vi "TDS RF Power Input Read.vi"(6 "Reference Level (dBm)":dbl, 8 "error in (no error)":errorcluster, 9 "Center Frequency (MHz)":dbl, 10 "Signal InstConfig":string, 11 "Address":string) -> (0 "error out":errorcluster, 3 "Power":dbl)   [LabVIEW 2025, in "Interface Functions.lvlib"]
uses:
  Interface Functions.lvlib
  <vilib>/Utility/error.llb/Trim Whitespace One-Sided.vi
  <instrlib>/Agilent U2000 Series/Agilent U2000 Series.lvlib
panel:
  out "Offset":dbl
  out "Commands":string[](array[string])
  # "RF Power Input Read"
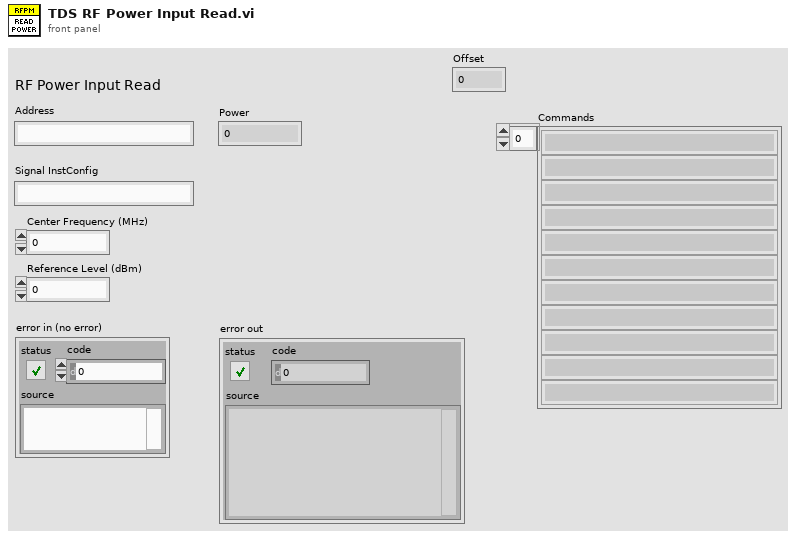
[diagram p1: front panel]
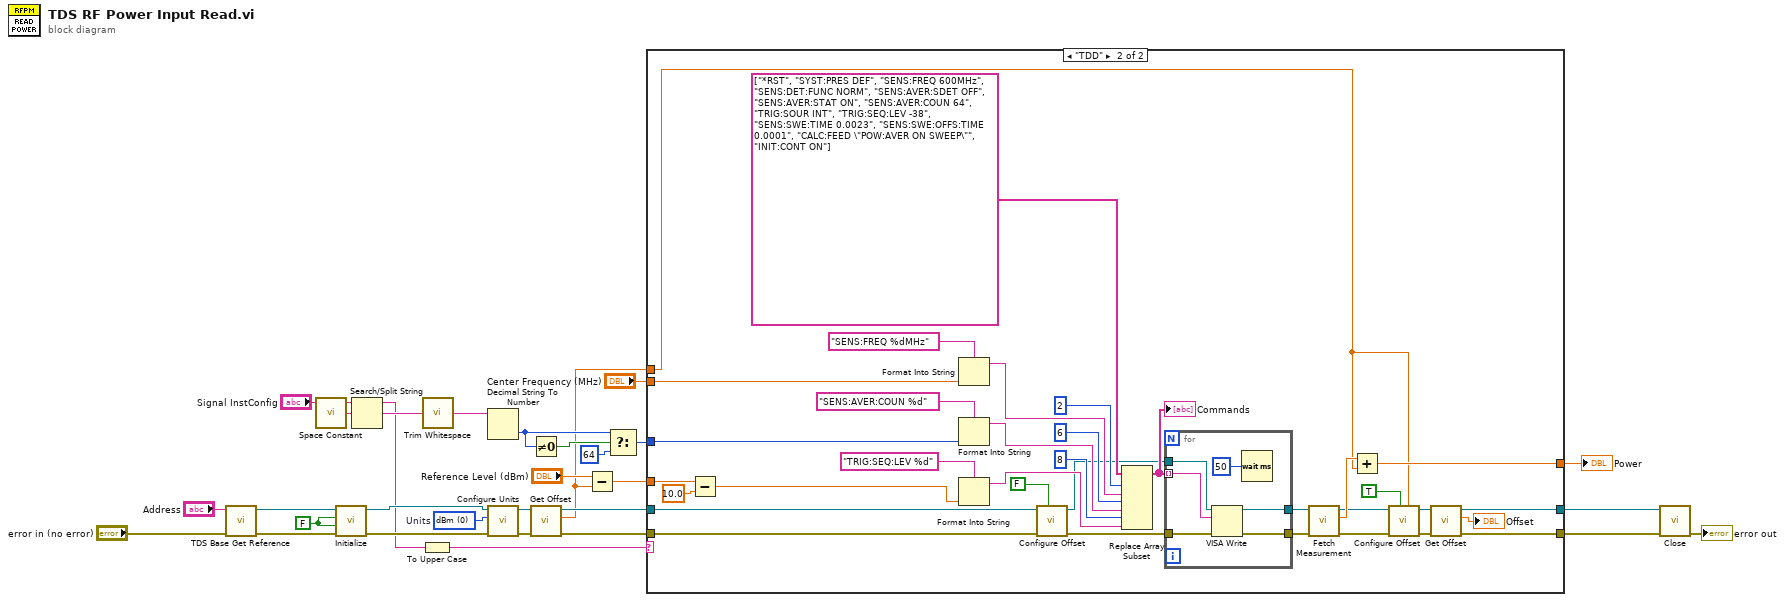
[diagram p0: block diagram]
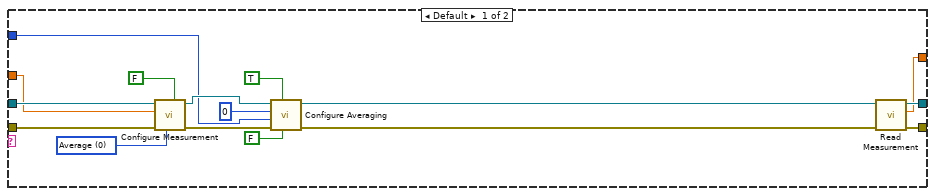
[diagram p2: hidden frame]
diagram:
  w17 = u16 0 items=["dBm", "W"]  # Units
  w19 = FALSE ("ID Query (True)")
  n1 = call "TDS Base Get Reference.vi"("error in (no error)"="error in (no error)", "Address"="Address") -> ("error out"=w25:errorcluster, "Reference"=w23:refnum<visa-resource-name>)  [unwired: 8 in]
  n2 = call <vilib>:"Space Constant.vi"() -> ("String"=w15:string)
  n3 = call <instrlib>:"Initialize.vi"("error in (no error)"=w25, "Reset (True)"=w19, "ID Query (True)"=w19, "VISA resource name"=w23) -> ("error out"=w18:errorcluster, "VISA resource name out"=w16:refnum<visa-resource-name>)  [unwired: 6 in]
  n4 = Search/Split String(string="Signal InstConfig", search string/char (-)=w15) -> (substring before match=w12:string, match + rest of string=w14:string)  [unwired: 1 in, 1 out]
  n5 = To Upper Case(1:w12) -> (0:w22:string)
  n6 = call <vilib>:"Trim Whitespace.vi"("string"=w14) -> ("trimmed string"=w13:string)  [unwired: 1 in]
  n7 = Decimal String To Number(string=w13) -> (number=w10:i32)  [unwired: 2 in, 1 out]
  n8 = call <instrlib>:"Configure Units.vi"("error in (no error)"=w18, "Units (0: dBm)"=w17, "VISA resource name"=w16) -> ("error out"=w6:errorcluster, "VISA resource name out"=w7:refnum<visa-resource-name>)  [unwired: 1 in, 6 out]
  n9 = Not Equal To 0?(x=w10) -> (x != 0?=w11:bool)
  n10 = call "Get Offset.vi"("error in (no error)"=w6, "VISA resource name"=w7) -> ("error out"=w5:errorcluster, "Offset"=w1:dbl, "VISA resource name out"=w4:refnum<visa-resource-name>)  [unwired: 7 in]
  n11 = Subtract(x="Reference Level (dBm)", y=w1) -> (x-y=w2:dbl)
  n12 = Select(t=w10, s=w11, f=64) -> (s? t:f=w8:i32)
  n13 = case shown="\"TDD\"" w22 {
    tunnel: [w41 w52] -> w21
    tunnel: [w42 w53] -> w20
    tunnel: [w40 w64] -> w26
    tunnel: w5 -> [w38 w60]
    tunnel: w2 -> [w35 w49]
    tunnel: "Center Frequency (MHz)" -> [_ w71]
    tunnel: w4 -> [w36 w62]
    tunnel: w8 -> [w31 w78]
    tunnel: w1 -> [_ w50]
    frame Default {
      w37 = 0 items=["Average", "Normal"] ("Measurement Function (0: Average)")
      n14 = call <instrlib>:"Configure Measurement.vi"("Enable Gate Feed (T: Enable)"=FALSE, "Measurement Function (0: Average)"=w37, "error in (no error)"=w38, "Expected Value (0)"=w35, "VISA resource name"=w36) -> ("error out"=w33:errorcluster, "VISA resource name out"=w34:refnum<visa-resource-name>)  [unwired: 5 in]
      n15 = call <instrlib>:"Configure Averaging.vi"("Auto Averaging (T: Enable)"=FALSE, "Enable Averaging (T: Enable)"=TRUE, "error in (no error)"=w33, "Averaging Count (4)"=w31, "Averaging Buffer Size (1)"=0, "VISA resource name"=w34) -> ("error out"=w44:errorcluster, "VISA resource name out"=w43:refnum<visa-resource-name>)  [unwired: 4 in]
      n16 = call <instrlib>:"Read Measurement.vi"("error in (no error)"=w44, "VISA resource name"=w43) -> ("error out"=w41:errorcluster, "Measurement"=w40:dbl, "VISA resource name out"=w42:refnum<visa-resource-name>)  [unwired: 7 in]
    }
    frame "TDD" {
      n17 = Subtract(x=w49, y=10.0) -> (x-y=w47:dbl)
      n18 = Format Into String(format string="SENS:FREQ %dMHz", w71) -> (resulting string=w68:string)  [unwired: 2 in, 1 out]
      n19 = Format Into String(format string="SENS:AVER:COUN %d", w78) -> (resulting string=w77:string)  [unwired: 2 in, 1 out]
      n20 = Format Into String(format string="TRIG:SEQ:LEV %d", w47) -> (resulting string=w74:string)  [unwired: 2 in, 1 out]
      n21 = call <instrlib>:"Configure Offset.vi"("Enable Offset (F: Disable)"=FALSE, "error in (no error)"=w60, "VISA resource name"=w62) -> ("error out"=w59:errorcluster, "VISA resource name out"=w61:refnum<visa-resource-name>)  [unwired: 7 in]
      n22 = Replace Array Subset(array=string[] ["*RST", "SYST:PRES DEF", "SENS:FREQ 600MHz", "SENS:DET:FUNC NORM", "SENS:AVER:SDET OFF", "SENS:AVER:STAT ON", "SENS:AVER:COUN 64", "TRIG:SOUR INT", "TRIG:SEQ:LEV -38", "SENS:SWE:TIME 0.0023", "SENS:SWE:OFFS:TIME 0.0001", "CALC:FEED \"POW:AVER ON SWEEP\"", "INIT:CONT ON"], new element #1=w68, index #1=2 ("index"), new element #2=w77, index #2=6 ("index"), new element #3=w74, index #3=8 ("index")) -> (w70:string[])
      "Commands" <- w70
      n23 = for {
        tunnel: w70 -> [w86] mode=indexing
        tunnel: [w85] -> w66
        tunnel: [w84] -> w67
        tunnel: w59 -> [w83]
        tunnel: w61 -> [w82]
        n24 = VISA Write(VISA resource name=w82, write buffer=w86, error in (no error)=w83) -> (VISA resource name out=w84:refnum<visa-resource-name>, error out=w85:errorcluster)  [unwired: 1 out]
        n25 = Wait (ms)(milliseconds to wait=u32 50) -> ()  [unwired: 1 out]
      }
      n26 = call <instrlib>:"Fetch Measurement.vi"("error in (no error)"=w66, "VISA resource name"=w67) -> ("error out"=w57:errorcluster, "Measurement"=w65:dbl, "VISA resource name out"=w58:refnum<visa-resource-name>)  [unwired: 7 in]
      n27 = Add(x=w65, y=w50) -> (x+y=w64:dbl)
      n28 = call <instrlib>:"Configure Offset.vi"("Offset Value (0 dB)"=w50, "Enable Offset (F: Disable)"=TRUE, "error in (no error)"=w57, "VISA resource name"=w58) -> ("error out"=w54:errorcluster, "VISA resource name out"=w55:refnum<visa-resource-name>)  [unwired: 6 in]
      n29 = call "Get Offset.vi"("error in (no error)"=w54, "VISA resource name"=w55) -> ("error out"=w52:errorcluster, "Offset"=→"Offset":dbl, "VISA resource name out"=w53:refnum<visa-resource-name>)  [unwired: 7 in]
    }
  }
  "Power" <- w26
  n30 = call <instrlib>:"Close.vi"("error in (no error)"=w21, "VISA resource name"=w20) -> ("error out"=→"error out":errorcluster)  [unwired: 9 in]
